vi "TDMS chan to HDF5 (str).vi"(0 "tdms file":refnum<k34>, 1 "close dataset? (T)":bool=TRUE, 5 "group name in":string, 7 "channel name in":string, 11 "error in (no error)":errorcluster, 13 "HDF5 Ref":T1) -> (4 "tdms file out":refnum<k34>, 6 "group name out":string, 8 "channel name out":string, 10 "dataset out":T1, 15 "error out":errorcluster)   [LabVIEW 2012]
uses:
  <vilib>/addons/_hdf5/library.llb/HDF5 Ref.ctl
  <vilib>/addons/_hdf5/dataspace.llb/H5S_seloper_t.ctl
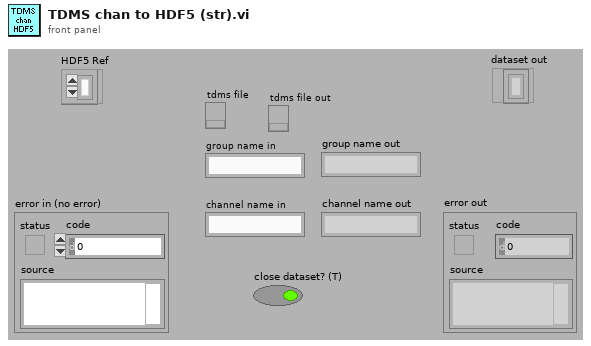
[diagram p1: front panel]
types:
  T1 = typedef "HDF5 Ref.ctl" = refnum<k1>
  T2 = typedef "H5S_seloper_t.ctl" = i32
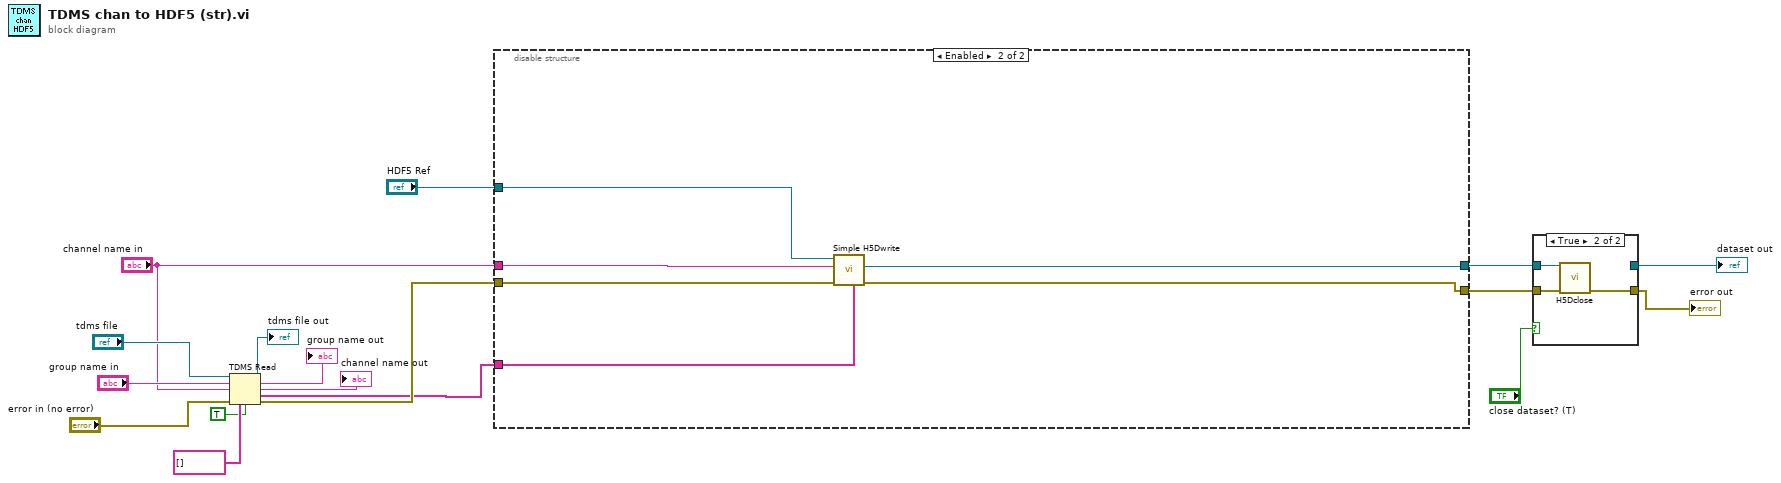
[diagram p0: block diagram]
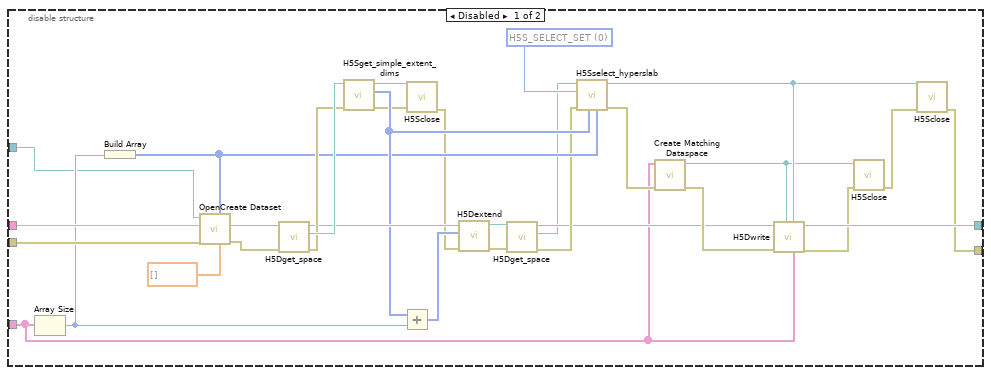
[diagram p2: hidden frame]
diagram:
  n1 = TDMS Read(0:"tdms file", 5:"group name in", 7:"channel name in", 11:"error in (no error)", 12:string[] [], 13:TRUE ("return channels in file order? (F)")) -> (4:→"tdms file out":refnum<k34>, 6:→"group name out":string, 8:→"channel name out":string, 10:w4:string[], 15:w13:errorcluster)  [unwired: 2 in, 1 out]
  n2 = disable-structure shown="Enabled" {
    disable-tunnel: "channel name in" -> [w48 w53]
    disable-tunnel: w13 -> [w47 w52]
    disable-tunnel: [w25 w50] -> w8
    disable-tunnel: [w19 w49] -> w7
    disable-tunnel: w4 -> [w24 w51]
    disable-tunnel: "HDF5 Ref" -> [w18 w54]
    frame Disabled {
      w41 = T2 0 items=["H5S_SELECT_NOOP"=-1, "H5S_SELECT_SET"=0, "H5S_SELECT_OR"=1, "H5S_SELECT_AND"=2, "H5S_SELECT_XOR"=3, "H5S_SELECT_NOTB"=4, "H5S_SELECT_NOTA"=5, "H5S_SELECT_APPEND"=6, "H5S_SELECT_PREPEND"=7] ("Operator")
      n3 = Array Size(array=w24) -> (size(s)=w35:i32)
      n4 = Build Array(w35) -> (w34:i32[])
      n5 = call "OpenCreate Dataset.vi"("Datatype"=dbl[] [], "Chunk size"=w34, "error in (no error)"=w47, "Dataset Path"=w48, "HDF5 Ref"=w18) -> ("error out"=w46:errorcluster, "HDF5 Dataset Ref out"=w38:T1)  [unwired: 4 in, 1 out]
      n6 = call <vilib>:"H5Dget_space.vi"("error in (no error)"=w46, "HDF5 Dataset Ref"=w38) -> ("error out"=w44:errorcluster, "HDF5 Dataspace Ref"=w45:T1, "HDF5 Dataset Ref out"=w42:T1)  [unwired: 5 in]
      n7 = call <vilib>:"H5Sget_simple_extent_dims.vi"("error in (no error)"=w44, "HDF5 Space Ref"=w45) -> ("error out"=w33:errorcluster, "Dims"=w40:i32[], "HDF5 Ref out"=w32:T1)  [unwired: 4 in, 1 out]
      n8 = Add(x=w40, y=w35) -> (x+y=w43:i32[])
      n9 = call <vilib>:"H5Sclose.vi"("error in (no error)"=w33, "HDF5 Dataspace Ref"=w32) -> ("error out"=w29:errorcluster)  [unwired: 7 in]
      n10 = call <vilib>:"H5Dextend.vi"("error in (no error)"=w29, "Size"=w43, "HDF5 Dataset Ref"=w42) -> ("error out"=w30:errorcluster, "HDF5 Dataset Ref out"=w31:T1)  [unwired: 5 in]
      n11 = call <vilib>:"H5Dget_space.vi"("error in (no error)"=w30, "HDF5 Dataset Ref"=w31) -> ("error out"=w28:errorcluster, "HDF5 Dataspace Ref"=w26:T1, "HDF5 Dataset Ref out"=w27:T1)  [unwired: 5 in]
      n12 = call <vilib>:"H5Sselect_hyperslab.vi"("Count"=w34, "Start"=w40, "error in (no error)"=w28, "Operator"=w41, "HDF5 Space Ref"=w26) -> ("error out"=w39:errorcluster, "HDF5 Ref out"=w22:T1)  [unwired: 5 in]
      n13 = call <vilib>:"Create Matching Dataspace.vi"("error in (no error)"=w39, "Data"=w24) -> ("error out"=w37:errorcluster, "HDF5 Dataspace Ref"=w21:T1)  [unwired: 6 in]
      n14 = call <vilib>:"H5Dwrite.vi"("Variant"=w24, "HDF5 File Space Ref (H5S_ALL)"=w22, "HDF5 Memory Space Ref (H5S_ALL)"=w21, "error in (no error)"=w37, "HDF5 Dataset Ref"=w27) -> ("error out"=w20:errorcluster, "HDF5 Ref out"=w25:T1)  [unwired: 5 in]
      n15 = call <vilib>:"H5Sclose.vi"("error in (no error)"=w20, "HDF5 Dataspace Ref"=w21) -> ("error out"=w23:errorcluster)  [unwired: 7 in]
      n16 = call <vilib>:"H5Sclose.vi"("error in (no error)"=w23, "HDF5 Dataspace Ref"=w22) -> ("error out"=w19:errorcluster)  [unwired: 7 in]
    }
    frame Enabled {
      n17 = call <vilib>:"Simple H5Dwrite.vi"("Data"=w51, "error in (no error)"=w52, "Dataset Path"=w53, "HDF5 Ref"=w54) -> ("error out"=w49:errorcluster, "HDF5 Dataset Ref out"=w50:T1)  [unwired: 5 in, 1 out]
    }
  }
  n18 = case shown="True" "close dataset? (T)" {
    tunnel: w8 -> [w56 w59]
    tunnel: w7 -> [w55 w58]
    tunnel: [w55 w57] -> w3
    tunnel: [w56 _] -> w5
    frame False {
    }
    frame True {
      n19 = call <vilib>:"H5Dclose.vi"("error in (no error)"=w58, "HDF5 Dataset Ref"=w59) -> ("error out"=w57:errorcluster)  [unwired: 7 in]
    }
  }
  "error out" <- w3
  "dataset out" <- w5
